vi "Connect.vi"(8 "error in (no error)":errorcluster, 9 "timeout":i32=-1, 11 "AF Queue Stream in":refnum<class "AF Queue Stream.lvclass">) -> (0 "error out":errorcluster, 3 "AF Queue Stream out":refnum<class "AF Queue Stream.lvclass">)   [LabVIEW 2020, in "AF Queue Stream.lvclass"]
doc: "Override this method to specify the action the local copy of this object will perform to connect to its remote counterpart."
uses:
  AF Queue Stream.lvclass
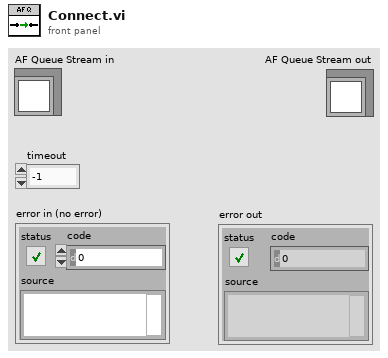
[diagram p1: front panel]
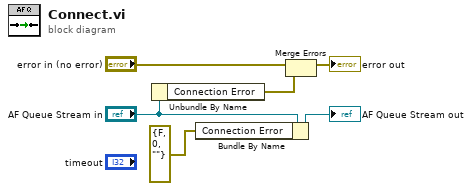
[diagram p0: block diagram]
diagram:
  n1 = Unbundle By Name("AF Queue Stream in") -> ("Connection Error"=w3:errorcluster)
  n2 = Bundle By Name(cluster="AF Queue Stream in", "Connection Error"=errorcluster {"status"=FALSE, "code"=0, "source"=""}) -> (→"AF Queue Stream out":refnum<class "AF Queue Stream.lvclass">)
  n3 = Merge Errors("error in (no error)", w3) -> (→"error out":errorcluster)
